vi "Process Image.vi"(8 "error in (no error)":errorcluster, 9 "session out":refnum<k35>, 10 "JSON string":string, 11 "Image in":T1) -> (0 "error out":errorcluster, 1 "session in":refnum<k35>, 2 "Color":i32, 3 "Image out":T1)   [LabVIEW 2020]
uses:
  <vilib>/vision/Image Controls.llb/IMAQ Image.ctl
  Controls/JSON image def.ctl
  <vilib>/vision/NI_Vision_Development_Module.lvlib
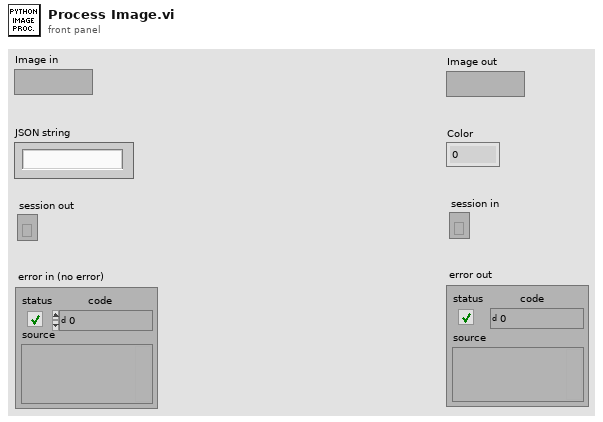
[diagram p1: front panel]
types:
  T1 = typedef "IMAQ Image.ctl" = refnum<image>
  T2 = typedef "JSON image def.ctl" = cluster{"Image Pixels (U8)":u8[][], "Image Pixels (U8) 2":u8[][], "Image Pixels (U8) 3":u8[][], "element":i32}
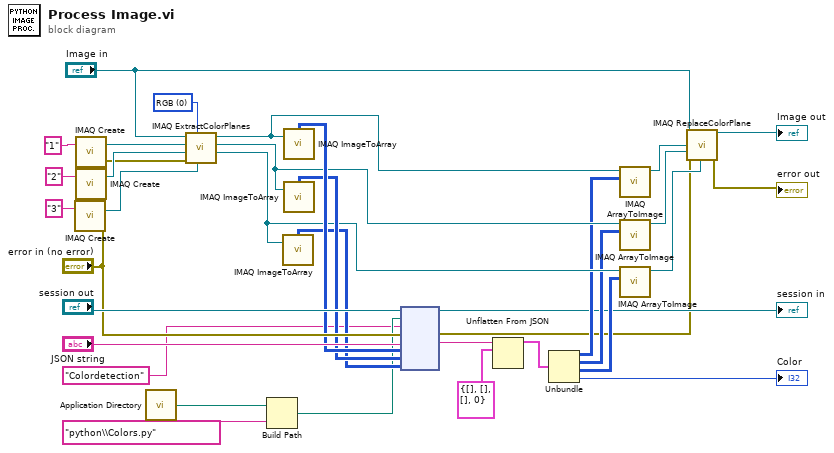
[diagram p0: block diagram]
diagram:
  w35 = u16 0 items=["RGB", "HSL", "HSV", "HSI"] ("Color Mode")
  n1 = call "IMAQ Create"("Image Name"="3") -> ("New Image"=w30:T1)  [unwired: 4 in, 1 out]
  n2 = call "IMAQ Create"("Image Name"="1") -> ("New Image"=w34:T1)  [unwired: 4 in, 1 out]
  n3 = call "IMAQ Create"("Image Name"="2") -> ("New Image"=w32:T1)  [unwired: 4 in, 1 out]
  n4 = call <vilib>:"Application Directory.vi"() -> ("Application Directory"=w22:path)
  n5 = call "IMAQ ExtractColorPlanes"("Blue or Luma or Val or Inten Plane"=w30, "Color Mode"=w35, "error in (no error)"="error in (no error)", "Green or Sat Plane"=w32, "Red or Hue Plane"=w34, "Image Src"="Image in") -> ("Blue or Luma or Val or Inten Plane out"=w14:T1, "Green or Sat Plane out"=w12:T1, "Red or Hue Plane out"=w10:T1)  [unwired: 2 in, 1 out]
  n6 = Build Path(base path=w22, name or relative path="python\\Colors.py") -> (appended path=w20:path)
  n7 = call "IMAQ ImageToArray"("Image"=w14) -> ("Image Pixels (U8)"=w23:u8[][])  [unwired: 3 in, 4 out]
  n8 = call "IMAQ ImageToArray"("Image"=w10) -> ("Image Pixels (U8)"=w25:u8[][])  [unwired: 3 in, 4 out]
  n9 = call "IMAQ ImageToArray"("Image"=w12) -> ("Image Pixels (U8)"=w24:u8[][])  [unwired: 3 in, 4 out]
  n10 = node("session out", w20, "Colordetection" ("function name"), "error in (no error)", "JSON string", w25, w24, w23) -> (→"session in":refnum<k35>, w4:errorcluster, w18:string)  [unwired: 3 in, 2 out]
  n11 = Unflatten From JSON(JSON string=w18, type and defaults=T2 {"Image Pixels (U8)"=[], "Image Pixels (U8) 2"=[], "Image Pixels (U8) 3"=[], "element"=0} ("anything")) -> (value=w16:T2)  [unwired: 5 in, 1 out]
  n12 = Unbundle(w16) -> ("Image Pixels (U8)"=w11:u8[][], "Image Pixels (U8) 2"=w13:u8[][], "Image Pixels (U8) 3"=w15:u8[][], "element"=→"Color":i32)
  n13 = call "IMAQ ArrayToImage"("Image Pixels (U8)"=w11, "Image"=w10) -> ("Image Out"=w7:T1)  [unwired: 8 in, 1 out]
  n14 = call "IMAQ ArrayToImage"("Image Pixels (U8)"=w13, "Image"=w12) -> ("Image Out"=w6:T1)  [unwired: 8 in, 1 out]
  n15 = call "IMAQ ArrayToImage"("Image Pixels (U8)"=w15, "Image"=w14) -> ("Image Out"=w5:T1)  [unwired: 8 in, 1 out]
  n16 = call "IMAQ ReplaceColorPlane"("Image Src"="Image in", "Red or Hue Plane"=w7, "Green or Sat Plane"=w6, "error in (no error)"=w4, "Blue or Luma or Val or Inten Plane"=w5) -> ("Image Dst Out"=→"Image out":T1, "error out"=→"error out":errorcluster)  [unwired: 9 in]
